vi "Set Sleep Mode.vi"(8 "error in (no error)":errorcluster, 10 "Sleep?":bool, 11 "PWM in":refnum<class "LINX-PCA9865 PWM.lvclass">) -> (0 "error out":errorcluster, 3 "PWM out":refnum<class "LINX-PCA9865 PWM.lvclass">)   [LabVIEW 2019, in "LINX-PCA9865 PWM.lvclass"]
uses:
  LINX-PCA9865 PWM.lvclass
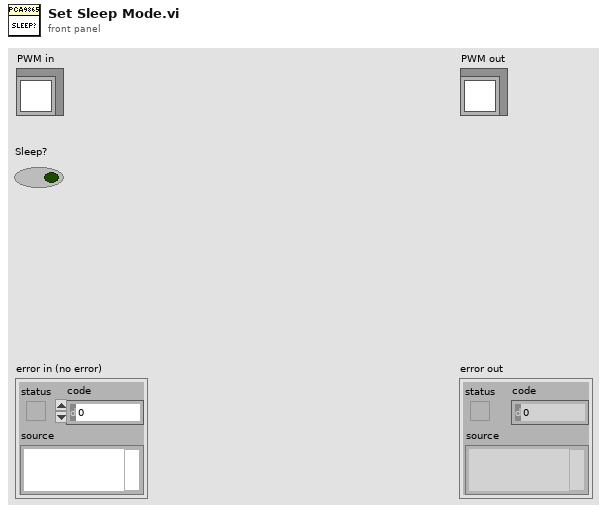
[diagram p1: front panel]
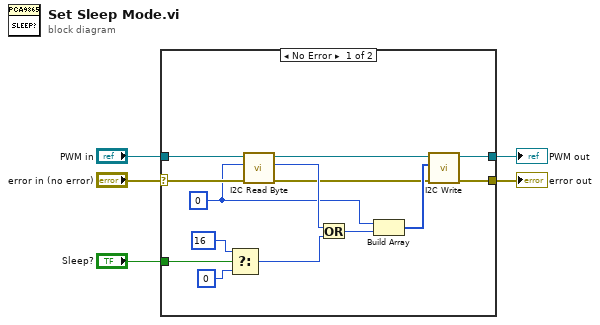
[diagram p0: block diagram]
diagram:
  n1 = case shown="No Error" "error in (no error)" {
    selector: "error in (no error)" -> [w18 w21]
    tunnel: [w10 w21] -> w4
    tunnel: [w11 w20] -> w2
    tunnel: "PWM in" -> [w19 w20]
    tunnel: "Sleep?" -> [w9 _]
    frame No Error {
      w13 = u8 0 ("Address")
      n2 = Select(t=u8 16 ("Address"), s=w9, f=u8 0 ("Address")) -> (s? t:f=w6:u8)
      n3 = call "I2C Read Byte.vi"("error in (no error)"=w18, "Address"=w13, "LINX-PCA9865 PWM in"=w19) -> ("error out"=w12:errorcluster, "Byte Read"=w16:u8, "LINX-PCA9865 PWM out"=w17:refnum<class "LINX-PCA9865 PWM.lvclass">)  [unwired: 6 in]
      n4 = Or(x=w16, y=w6) -> (x .or. y?=w15:u8)
      n5 = Build Array(w13, w15) -> (w14:u8[])
      n6 = call "I2C Write.vi"("error in (no error)"=w12, "Bytes to Write"=w14, "LINX-PCA9865 PWM in"=w17) -> ("error out"=w10:errorcluster, "LINX-PCA9865 PWM out"=w11:refnum<class "LINX-PCA9865 PWM.lvclass">)  [unwired: 7 in]
    }
    frame Error {
    }
  }
  "error out" <- w4
  "PWM out" <- w2
